vi "Low Threshold with Hysteresis.vi"(0 "Alt Dif":dbl(slide)=302.3255813953488 scale=-1000.0..1000.0, 1 "Reset":bool, 2 "Threshold":dbl=-50.0, 3 "Hysteresis":dbl=200.0) -> (5 "Boolean":bool, 6 "Peak":dbl=4.0)   [LabVIEW 2012]
doc: "Use this template to build a standard state machine design pattern. Each state executes code and determines which state to transition to. Contrast this design pattern with the User Interface Event Handler pattern, in which code executes in response to user actions. Contrast this design pattern also with the Queued Message Handler pattern, in which each message handling code can queue zero or more new messages."
uses:
  peak w hysteresis.ctl
panel:
  out "comparator":dbl=-302.3255813953488
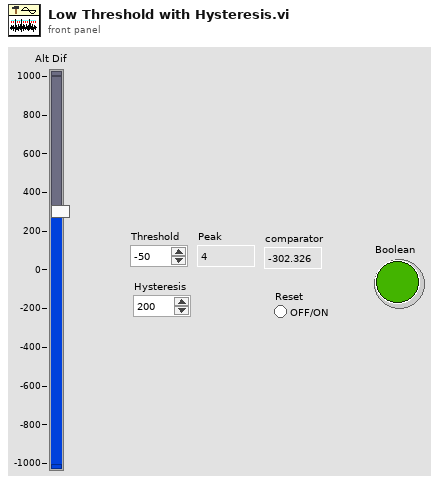
[diagram p1: front panel]
types:
  T1 = typedef "peak w hysteresis.ctl" = enum16{"Wait", "Peak", "Repeat?", "Stop"}
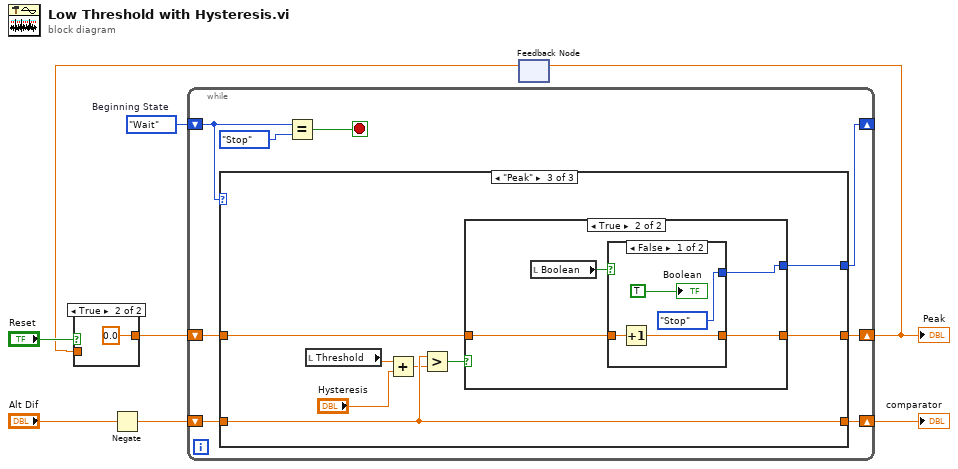
[diagram p0: block diagram]
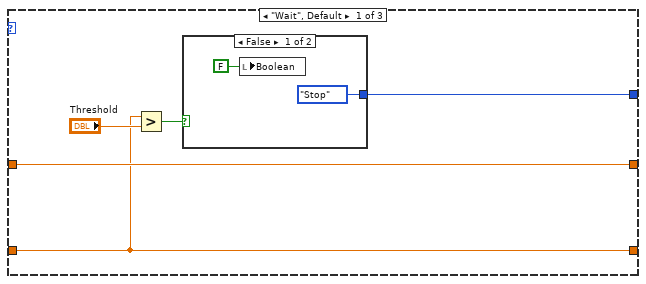
[diagram p3: hidden frame]
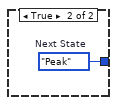
[diagram p4: hidden frame]
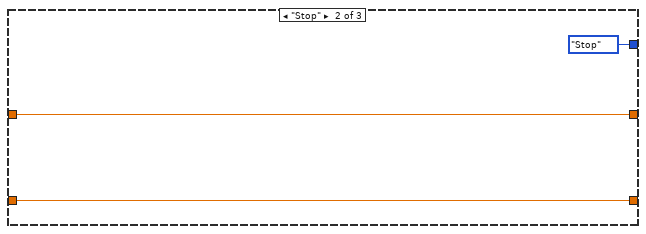
[diagram p5: hidden frame]
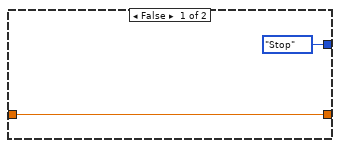
[diagram p6: hidden frame]
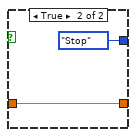
[diagram p7: hidden frame]
diagram:
  w8 = peak_w_hysteresis."Wait"  # Beginning State
  n1 = Negate(x="Alt Dif") -> (-x=w1:dbl)
  n2 = feedback #1() -> (w2:dbl)  [unwired: 1 in]
  n3 = case shown="True" "Reset" {
    tunnel: [w9 0.0] -> w6
    tunnel: w2 -> [w9 _]
    frame False {
    }
    frame True {
    }
  }
  n4 = while {
    shift-right: [w15] -> _
    shift-left: w8 -> [w16]
    shift-right: [w11] -> w7
    shift-left: w1 -> [w14]
    shift-right: [w12] -> w3
    shift-left: w6 -> [w13]
    stop <- w18 stop-if-true
    n5 = case shown="\"Peak\"" w16 {
      tunnel: [w23 peak_w_hysteresis."Stop" ("Next State") w34] -> w15
      tunnel: w14 -> [w19 w28 w35]
      tunnel: [w19 w28 w35] -> w11
      tunnel: w13 -> [w20 w27 w37]
      tunnel: [w20 w27 w36] -> w12
      frame "Wait", Default {
        n6 = Greater?(x=w19, y="Threshold") -> (0:w22:bool)
        n7 = case shown="False" w22 {
          tunnel: [peak_w_hysteresis."Stop" ("Next State") w26] -> w23
          frame False {
            n8 = local write "Boolean"(FALSE ("Boolean")) -> ()
          }
          frame True {
            w26 = peak_w_hysteresis."Peak"  # Next State
          }
        }
      }
      frame "Stop" {
      }
      frame "Peak" {
        n9 = local read "Threshold"() -> (w31:dbl)
        n10 = Add(x=w31, y="Hysteresis") -> (x+y=w32:dbl)
        n11 = Greater?(x=w35, y=w32) -> (0:w33:bool)
        n12 = case shown="True" w33 {
          tunnel: w37 -> [w39 w43]
          tunnel: [w39 w42] -> w36
          tunnel: [peak_w_hysteresis."Stop" ("Next State") w41] -> w34
          frame False {
          }
          frame True {
            n13 = local read "Boolean"() -> (w40:bool)
            n14 = case shown="False" w40 {
              tunnel: w43 -> [w46 w48]
              tunnel: [w45 w48] -> w42
              tunnel: [peak_w_hysteresis."Stop" ("Next State") peak_w_hysteresis."Stop" ("Next State")] -> w41
              frame False {
                n15 = Increment(x=w46) -> (x+1=w45:dbl)
                "Boolean" <- TRUE ("Boolean")
              }
              frame True {
              }
            }
          }
        }
      }
    }
    n16 = Equal?(x=w16, y=peak_w_hysteresis."Stop" ("States")) -> (x = y?=w18:bool)
  }
  "Peak" <- w3
  "comparator" <- w7
  n17 = feedback-in #1(w3) -> ()
